vi "EdgeDetection.vi"(7 "Boolean":bool) -> (8 "Boolean 2":bool)   [LabVIEW 2018]
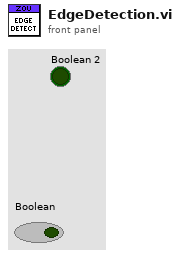
[diagram p1: front panel]
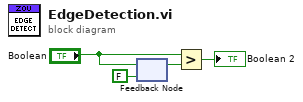
[diagram p0: block diagram]
diagram:
  n1 = feedback-in #1("Boolean") -> ()
  n2 = feedback #1(FALSE ("Boolean")) -> (w3:bool)
  n3 = Greater?(x="Boolean", y=w3) -> (0:→"Boolean 2":bool)
